vi "LauncherAngleTalon.vi"() -> ()   [LabVIEW 2012]
uses:
  State_Machine_Enum.ctl
  Robot Global Data.vi
panel:
  in  "Start at bottom?":bool=TRUE
  in  "Tolerance":dbl=0.05
  in  "LSBackwardValue":dbl=-0.4 min=-1.0 max=0.0 step=0.1
  in  "LSForwardValue":dbl=0.40000000000000013 min=0.0 max=1.0 step=0.1
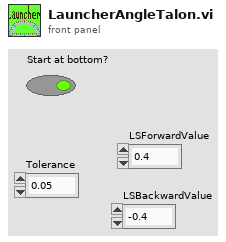
[diagram p1: front panel]
types:
  T1 = typedef "State_Machine_Enum.ctl" = enum16{"Idle", "Start", "Do", "Stop", "Init"}
  T2 = typedef "LoopDisable.ctl" = cluster{"Climb.vi":bool, "LauncherAngle.vi":bool, "Launcher.vi":bool, "ArmControl.vi":bool, "WinchMotor.vi":bool, "ReadDriveEncoder.vi":bool}
  T3 = typedef "WPI_DigitalInputDevRef.ctl" = cluster{"DevStatus":errorcluster, "DIO Channel":T4, "Digital Module":T5}
  T4 = typedef "FPGA_DIOChannel.ctl" = enum8{"DIO 1", "DIO 2", "DIO 3", "DIO 4", "DIO 5", "DIO 6", "DIO 7", "DIO 8", "DIO 9", "DIO 10", "DIO 11", "DIO 12", "DIO 13", "DIO 14", "Invalid"}
  T5 = typedef "FPGA_TypedefDigitalModule.ctl" = enum16{"Digital Module 1", "Digital Module 2"}
  T6 = typedef "WPI_EncoderDevRef.ctl" = cluster{"DevStatus":errorcluster, "EncoderIndex":T7, "CounterIndex":T8, "DistancePerCount":dbl, "Decoding Type":T9}
  T7 = typedef "FPGA_EncoderIdx.ctl" = enum8{"Enc 0", "Enc 1", "Enc 2", "Enc 3", "Invalid"}
  T8 = typedef "FPGA_CounterCtrSystemIndex.ctl" = enum8{"Ctr 0", "Ctr 1", "Ctr 2", "Ctr 3", "Ctr 4", "Ctr 5", "Ctr 6", "Ctr 7", "Invalid"}
  T9 = typedef "WPI_EncoderType.ctl" = enum16{"1x", "2x", "4x"}
  T10 = typedef "WPI_MotorControlDeviceRef.ctl" = cluster{"DeviceStatus":errorcluster, "Type":enum16{"PWM", "CAN"}, "PWM":cluster{"Digital Module":T5, "PWM Channel":T11, "DeadBand":T12}, "CAN":cluster{"Device Number":u8, "Control Mode":T13, "Semaphore":T14, "Max Vout":dbl}, "Invert":bool, "TransformRef":T15, "InvTransformRef":T15}
  T11 = typedef "FPGA_DIOPWMChannel.ctl" = enum8{"PWM 1", "PWM 2", "PWM 3", "PWM 4", "PWM 5", "PWM 6", "PWM 7", "PWM 8", "PWM 9", "PWM 10", "Invalid"}
  T12 = typedef "WPI_PWMDeadband.ctl" = cluster{"Name":string, "maxPositivePwm":i32, "minPositivePwm":i32, "centerPwm":i32, "maxNegativePwm":i32, "minNegativePwm":i32, "angularRange":u16}
  T13 = typedef "WPI_CANJaguar_ControlMode.ctl" = enum8{"Percent VBus", "Current", "Speed", "Position", "Voltage"}
  T14 = typedef "Semaphore RefNum" = refnum<k1>
  T15 = typedef "WPI_PWMTransform_ConPane.ctl" = refnum<vi>
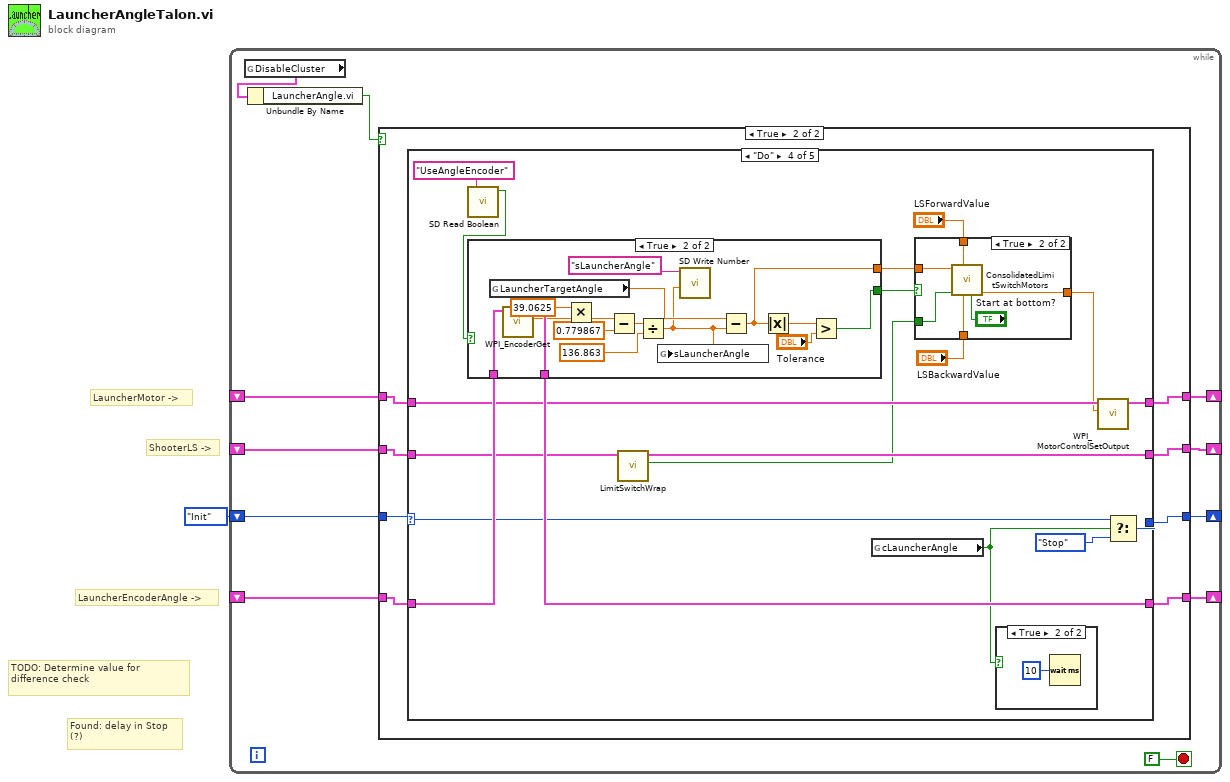
[diagram p0: block diagram]
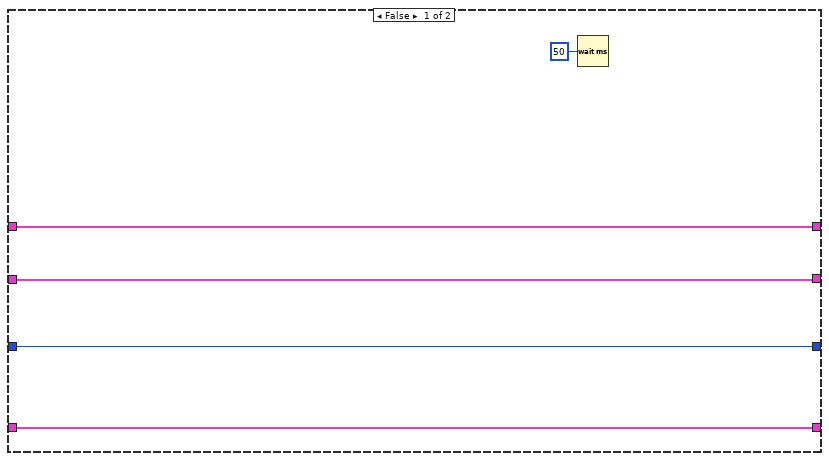
[diagram p2: hidden frame]
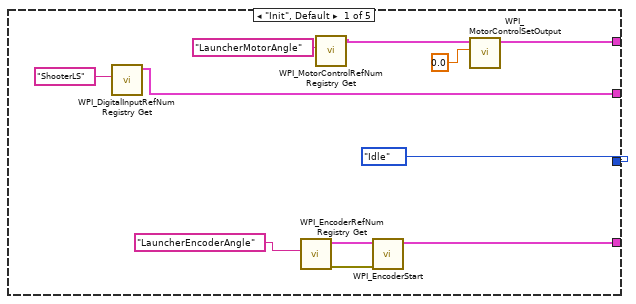
[diagram p3: hidden frame]
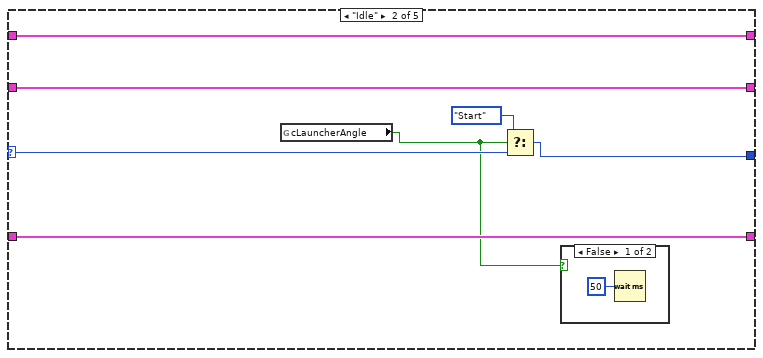
[diagram p4: hidden frame]
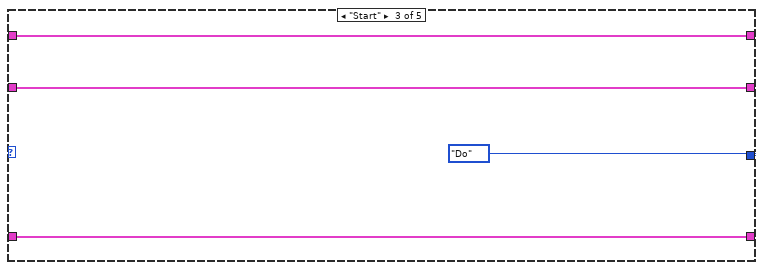
[diagram p6: hidden frame]
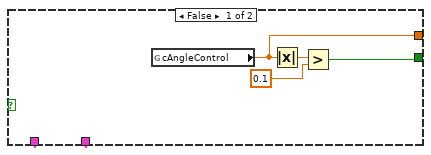
[diagram p7: hidden frame]
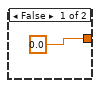
[diagram p9: hidden frame]
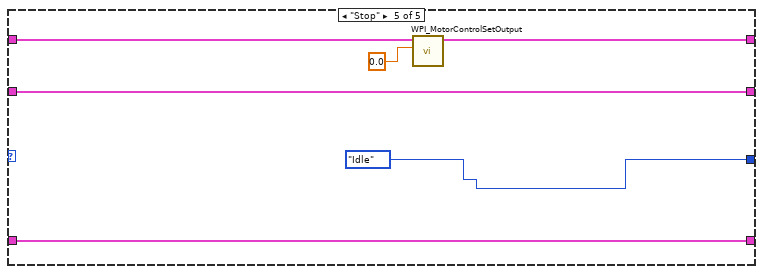
[diagram p10: hidden frame]
diagram:
  # "ShooterLS ->"
  # "Found: delay in Stop \n(?)"
  # "TODO: Determine value for difference check"
  # "LauncherEncoderAngle ->"
  # "LauncherMotor ->"
  n1 = while {
    shift-right: [w10] -> _
    shift-left: State_Machine_Enum."Init" ("State") -> [w11]
    shift-right: [w9] -> _
    shift-left: _ -> [w8]
    shift-right: [w4] -> _
    shift-left: _ -> [w3]
    shift-right: [w6] -> _
    shift-left: _ -> [w7]
    stop <- FALSE stop-if-true
    n2 = global read "Robot Global Data.vi" "DisableCluster"() -> (w5:T2)
    n3 = Unbundle By Name(w5) -> ("LauncherAngle.vi"=w2:bool)
    n4 = case shown="True" w2 {
      tunnel: w11 -> [w16 w25]
      tunnel: [w16 w24] -> w10
      tunnel: [w15 w23] -> w9
      tunnel: w8 -> [w15 w22]
      tunnel: w7 -> [w17 w21]
      tunnel: [w17 w20] -> w6
      tunnel: [w13 w19] -> w4
      tunnel: w3 -> [w13 w18]
      frame False {
        n5 = Wait (ms)(milliseconds to wait=u32 50) -> ()  [unwired: 1 out]
      }
      frame True {
        n6 = case shown="\"Do\"" w25 {
          selector: w25 -> [_ w41 _ w63 _]
          tunnel: [State_Machine_Enum."Idle" ("State") w42 State_Machine_Enum."Do" ("State") w62 State_Machine_Enum."Idle" ("State")] -> w24
          tunnel: [w33 w39 w47 w64 w100] -> w23
          tunnel: w22 -> [_ w39 w47 w65 w100]
          tunnel: w21 -> [_ w40 w46 w51 w99]
          tunnel: [w30 w40 w46 w50 w99] -> w20
          tunnel: [w29 w37 w45 w57 w97] -> w19
          tunnel: w18 -> [_ w37 w45 w58 w98]
          frame "Init", Default {
            n7 = call <vilib>:"WPI_DigitalInputRefNum Registry Get.vi"("refnum name"="ShooterLS") -> ("DigitalInputDevRef"=w30:T3)  [unwired: 9 in, 1 out]
            n8 = call <vilib>:"WPI_EncoderRefNum Registry Get.vi"("refnum name"="LauncherEncoderAngle") -> ("error out"=w32:errorcluster, "EncoderDevRef"=w34:T6)  [unwired: 9 in]
            n9 = call <vilib>:"WPI_MotorControlRefNum Registry Get.vi"("refnum name"="LauncherMotorAngle") -> ("MotorControlDevRef"=w27:T10)  [unwired: 9 in, 1 out]
            n10 = call <vilib>:"WPI_EncoderStart.vi"("error in (no error)"=w32, "EncoderDevRef"=w34) -> ("EncoderDevRef"=w33:T6)  [unwired: 8 in, 1 out]
            n11 = call <vilib>:"WPI_MotorControlSetOutput.vi"("Output"=0.0, "MotorControlDevRef"=w27) -> ("MotorControlDevRef"=w29:T10)  [unwired: 7 in, 2 out]
          }
          frame "Idle" {
            n12 = global read "Robot Global Data.vi" "cLauncherAngle"() -> (w38:bool)
            n13 = Select(t=State_Machine_Enum."Start" ("State"), s=w38, f=w41) -> (s? t:f=w42:T1)
            n14 = case shown="False" w38 {
              frame False {
                n15 = Wait (ms)(milliseconds to wait=u32 50) -> ()  [unwired: 1 out]
              }
              frame True {
              }
            }
          }
          frame "Start" {
          }
          frame "Do" {
            n16 = call <vilib>:"SD Read Boolean.vi"("Name"="UseAngleEncoder") -> ("Boolean"=w52:bool)  [unwired: 8 in, 2 out]
            n17 = case shown="True" w52 {
              tunnel: w65 -> [w67 w86]
              tunnel: [w67 w85] -> w64
              tunnel: [w68 w82] -> w61
              tunnel: [w69 w81] -> w60
              frame False {
                n18 = global read "Robot Global Data.vi" "cAngleControl"() -> (w68:dbl)
                n19 = Absolute Value(x=w68) -> (abs(x)=w71:dbl)
                n20 = Greater?(x=w71, y=0.1) -> (0:w69:bool)
              }
              frame True {
                n21 = global read "Robot Global Data.vi" "LauncherTargetAngle"() -> (w77:dbl)
                n22 = call <vilib>:"WPI_EncoderGet.vi"("EncoderDevRef"=w86) -> ("Distance"=w73:dbl, "EncoderDevRef"=w85:T6)  [unwired: 5 in, 4 out]
                n23 = Multiply(x=39.0625, y=w73) -> (x*y=w74:dbl)
                n24 = Subtract(x=w74, y=0.779867) -> (x-y=w80:dbl)
                n25 = Divide(x=w80, y=136.863) -> (x/y=w76:dbl)
                n26 = global write "Robot Global Data.vi" "sLauncherAngle"(w76) -> ()
                n27 = call <vilib>:"SD Write Number.vi"("Numeric"=w76, "Name"="sLauncherAngle") -> ()  [unwired: 8 in, 2 out]
                n28 = Subtract(x=w77, y=w76) -> (x-y=w82:dbl)
                n29 = Absolute Value(x=w82) -> (abs(x)=w84:dbl)
                n30 = Greater?(x=w84, y="Tolerance") -> (0:w81:bool)
              }
            }
            n31 = call "LimitSwitchWrap.vi"("DigitalInputDevRef"=w51) -> ("Triggered"=w49:bool, "DigitalInputDevRef 2"=w50:T3)  [unwired: 9 in]
            n32 = global read "Robot Global Data.vi" "cLauncherAngle"() -> (w59:bool)
            n33 = case shown="True" w60 {
              tunnel: w61 -> [_ w90]
              tunnel: [0.0 ("New Output") w94] -> w54
              tunnel: w49 -> [_ w93]
              tunnel: "LSBackwardValue" -> [_ w92]
              tunnel: "LSForwardValue" -> [_ w91]
              frame False {
              }
              frame True {
                n34 = call "ConsolidatedLimitSwitchMotors.vi"("Start at bottom?"="Start at bottom?", "BackwardValue"=w92, "ForwardValue"=w91, "CurrentLSValue"=w93, "CurrentInput"=w90) -> ("New Output"=w94:dbl)  [unwired: 6 in]
              }
            }
            n35 = case shown="True" w59 {
              frame False {
              }
              frame True {
                n36 = Wait (ms)(milliseconds to wait=u32 10) -> ()  [unwired: 1 out]
              }
            }
            n37 = call <vilib>:"WPI_MotorControlSetOutput.vi"("Output"=w54, "MotorControlDevRef"=w58) -> ("MotorControlDevRef"=w57:T10)  [unwired: 7 in, 2 out]
            n38 = Select(t=w63, s=w59, f=State_Machine_Enum."Stop" ("State")) -> (s? t:f=w62:T1)
          }
          frame "Stop" {
            n39 = call <vilib>:"WPI_MotorControlSetOutput.vi"("Output"=0.0, "MotorControlDevRef"=w98) -> ("MotorControlDevRef"=w97:T10)  [unwired: 7 in, 2 out]
          }
        }
      }
    }
  }
